vi "FITS_Test_Read_Keyword.vi"() -> ()   [LabVIEW 2016]
panel:
  out "Record":string
  in  "Keyword to Read":string="BITPIX"
  out "error out":errorcluster
  in  "Path":path=path "/home/shrc/HRCSoft/modules/FITS/test/fits_test.fits"
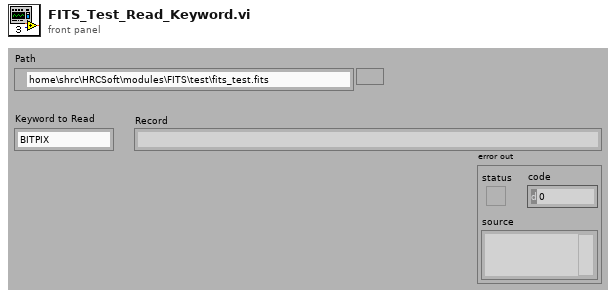
[diagram p1: front panel]
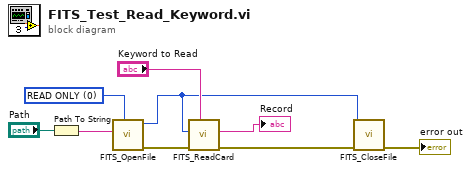
[diagram p0: block diagram]
diagram:
  w7 = 0 items=["READ ONLY", "READ/WRITE"] ("mode")
  n1 = Path To String(path="Path") -> (string=w8:string)
  n2 = call "FITS_OpenFile.vi"("mode"=w7, "filename"=w8) -> ("error out"=w5:errorcluster, "fp out"=w1:u32)  [unwired: 1 in, 7 out]
  n3 = call "FITS_ReadCard.vi"("Keyname"="Keyword to Read", "error in"=w5, "ref"=w1) -> ("error out"=w4:errorcluster, "Record"=→"Record":string)  [unwired: 7 out]
  n4 = call "FITS_CloseFile.vi"("error in"=w4, "ref"=w1) -> ("error out"=→"error out":errorcluster)  [unwired: 9 out]
